vi "Deactivate-selected-motors.vi"(8 "error in (no error)":errorcluster, 10 "Selected motors":T1, 11 "Available motors in":refnum<class "Motor-assembly.lvclass">) -> (0 "error out":errorcluster, 3 "Available motors out":refnum<class "Motor-assembly.lvclass">)   [LabVIEW 2013, in "PowderDeposition.lvlib" / "Motor-assembly.lvclass"]
doc: "Deactivate the motors that are selected - correspondig button pressed - but not yet active."
uses:
  Motor-assembly.lvclass
  Motor-selection.ctl
  Motor/Motor.lvclass
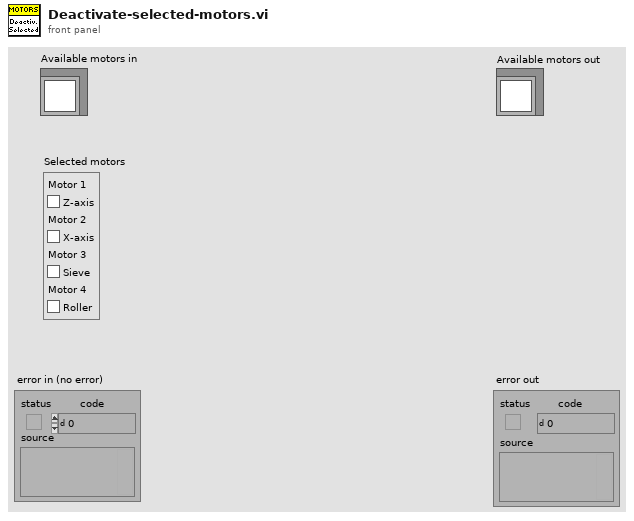
[diagram p1: front panel]
types:
  T1 = typedef "PowderDeposition.lvlib/Motor-assembly.lvclass/Motor-selection.ctl" = cluster{"Motor 1":bool, "Motor 2":bool, "Motor 3":bool, "Motor 4":bool}
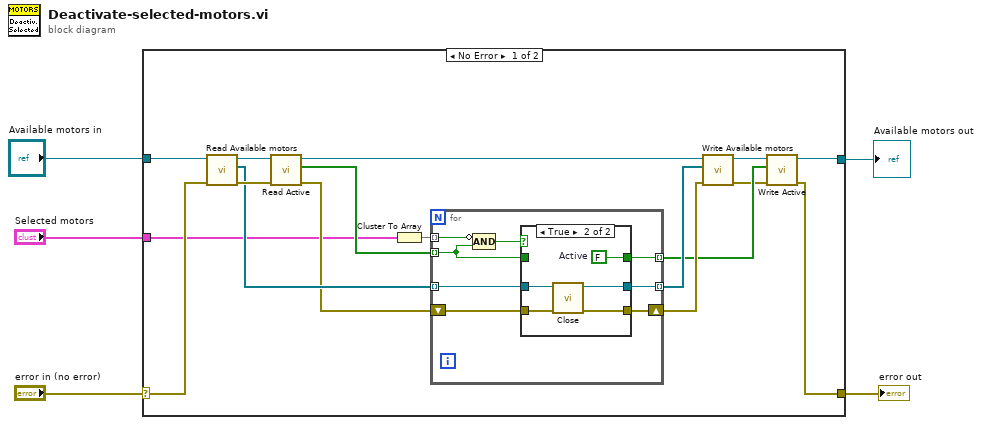
[diagram p0: block diagram]
diagram:
  n1 = case shown="No Error" "error in (no error)" {
    selector: "error in (no error)" -> [w22 w40]
    tunnel: [w6 w40] -> w4
    tunnel: "Available motors in" -> [w9 w39]
    tunnel: [w8 w39] -> w2
    tunnel: "Selected motors" -> [w7 _]
    frame No Error {
      n2 = call-dynamic "Read Available motors.vi"("error in (no error)"=w22, "Available motors in"=w9) -> ("error out"=w20:errorcluster, "Available motors"=w17:refnum<class "Motor.lvclass">[], "Available motors out"=w21:refnum<class "Motor-assembly.lvclass">)  [unwired: 7 in]
      n3 = call-dynamic "Read Active.vi"("error in (no error)"=w20, "Available motors in"=w21) -> ("error out"=w16:errorcluster, "Active?"=w18:bool[], "Available motors out"=w13:refnum<class "Motor-assembly.lvclass">)  [unwired: 7 in]
      n4 = Cluster To Array(cluster=w7) -> (array=w19:bool[])
      n5 = for {
        tunnel: w19 -> [w30] mode=indexing
        tunnel: w18 -> [w24] mode=indexing
        tunnel: w17 -> [w28] mode=indexing
        tunnel: [w27] -> w14 mode=indexing
        shift-right: [w25] -> w15
        shift-left: w16 -> [w26]
        tunnel: [w23] -> w12 mode=indexing
        n6 = Compound Arithmetic op=AND(invert w30, w24) -> (w29:bool)
        n7 = case shown="True" w29 {
          tunnel: w28 -> [w33 w38]
          tunnel: [w33 w37] -> w27
          tunnel: w26 -> [w32 w36]
          tunnel: [w32 w35] -> w25
          tunnel: w24 -> [w31 _]
          tunnel: [w31 w34] -> w23
          frame False {
          }
          frame True {
            w34 = FALSE  # Active
            n8 = call-dynamic "Close.vi"("error in (no error)"=w36, "Motor in"=w38) -> ("error out"=w35:errorcluster, "Motor out"=w37:refnum<class "Motor.lvclass">)  [unwired: 8 in]
          }
        }
      }
      n9 = call-dynamic "Write Available motors.vi"("error in (no error)"=w15, "Available motors"=w14, "Available motors in"=w13) -> ("error out"=w10:errorcluster, "Available motors out"=w11:refnum<class "Motor-assembly.lvclass">)  [unwired: 7 in]
      n10 = call-dynamic "Write Active.vi"("error in (no error)"=w10, "Active?"=w12, "Available motors in"=w11) -> ("error out"=w6:errorcluster, "Available motors out"=w8:refnum<class "Motor-assembly.lvclass">)  [unwired: 7 in]
    }
    frame Error {
    }
  }
  "error out" <- w4
  "Available motors out" <- w2
